vi "Scheduler_Cluster.vi"() -> ()   [LabVIEW 2014]
panel:
  in  "Numeric":i32=50
  out "Waveform Chart":i32(graph)
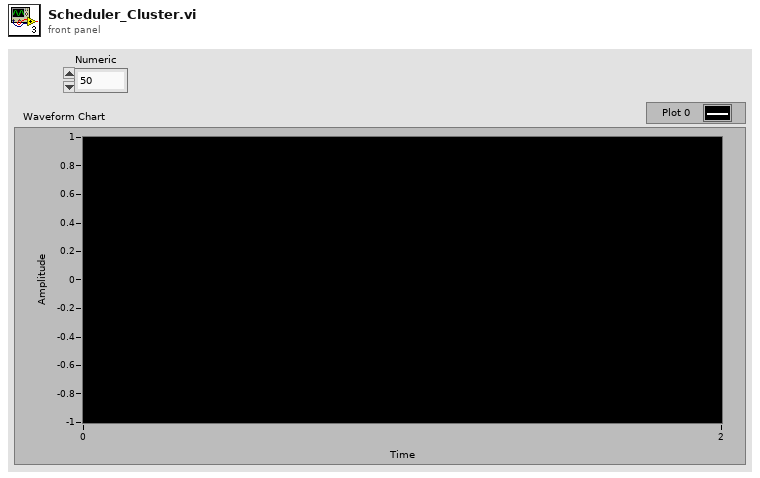
[diagram p1: front panel]
types:
  T1 = cluster{"number: 0 to 1":dbl, "number: 0 to 1":dbl, "number: 0 to 2":dbl}
  T2 = cluster{"number: 0 to 1":dbl, "number: 0 to 1":dbl}
  T3 = cluster{"number: 0 to 1":dbl, "number: 0 to 1":dbl, "number: 0 to 1":dbl}
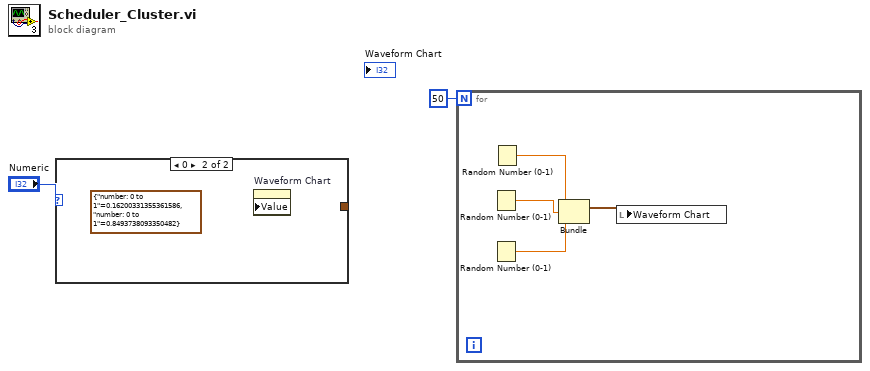
[diagram p0: block diagram]
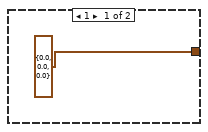
[diagram p2: hidden frame]
diagram:
  n1 = case shown="0" "Numeric" {
    tunnel: [T1 {"number: 0 to 1"=0.0, "number: 0 to 1"=0.0, "number: 0 to 2"=0.0} ("Waveform Chart") _] -> _
    frame 1 {
    }
    frame 0 {
      (unwired) T2 {"number: 0 to 1"=0.16200331355361586, "number: 0 to 1"=0.8493738093350482} ("Waveform Chart")
      n2 = property on="Waveform Chart" class="WFChart (strict)" props=["Value"]() -> ()  [unwired: 3 in, 2 out]
    }
  }
  n3 = for {
    N: 50 -> [_]
    n4 = Random Number (0-1)() -> (number: 0 to 1=w6:dbl)
    n5 = Random Number (0-1)() -> (number: 0 to 1=w5:dbl)
    n6 = Random Number (0-1)() -> (number: 0 to 1=w7:dbl)
    n7 = Bundle("number: 0 to 1"=w7, "number: 0 to 1"=w6, "number: 0 to 1"=w5) -> (w4:T3)  [unwired: 1 in]
    n8 = local write "Waveform Chart"(w4) -> ()
  }
